vi "TCL Get Fragments - Nevent1frag.vi"(0 "event file":path, 1 "event numbers":i32[](array[numeric]), 3 "primary key":string, 4 "fragment":string, 5 "error in (no error)":errorcluster) -> (6 "fragments out":string[](array[string]), 7 "values":string[][](array[string]), 8 "error out":errorcluster)   [LabVIEW 2010]
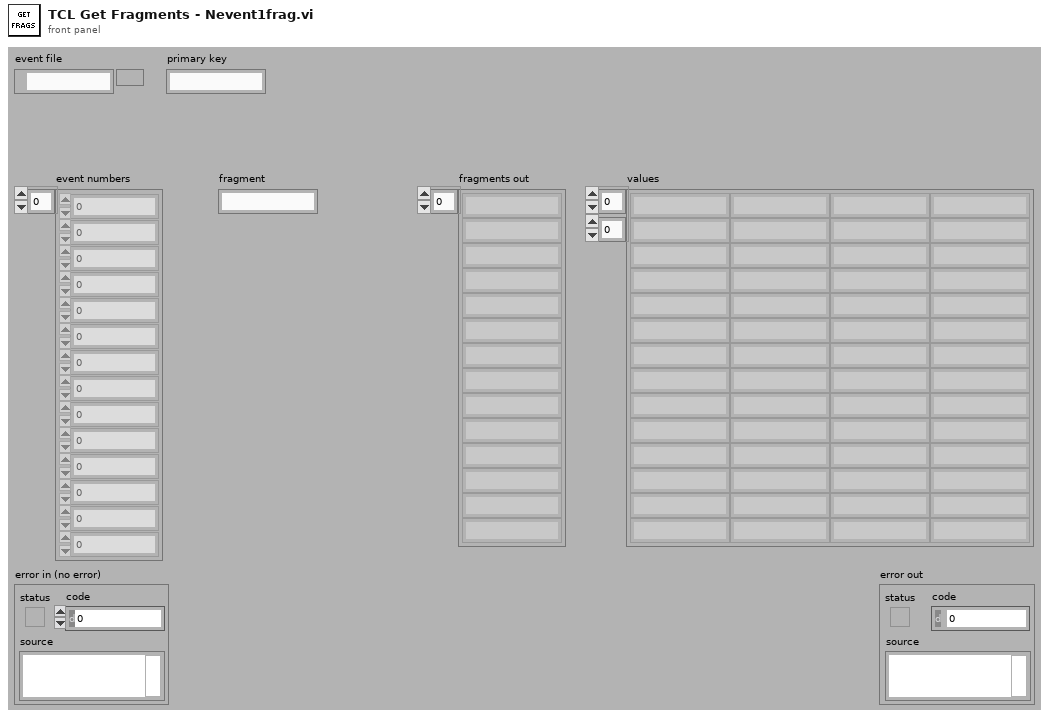
[diagram p1: front panel]
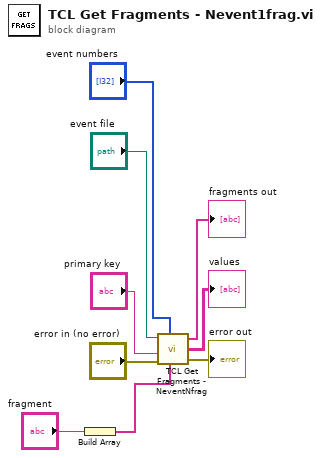
[diagram p0: block diagram]
diagram:
  n1 = Build Array("fragment") -> (w4:string[])
  n2 = call "TCL Get Fragments - NeventNfrag.vi"("event file"="event file", "event numbers"="event numbers", "primary key"="primary key", "fragments"=w4, "error in (no error)"="error in (no error)") -> ("fragments out"=→"fragments out":string[], "values"=→"values":string[][], "error out"=→"error out":errorcluster)  [unwired: 1 in]
